vi "SetCellValuesInXLS.vi"() -> ()   [LabVIEW 2013]
uses:
  C:/PhaeronGit/LVNPOI/Resources/NPOI 2.1.1 dotnet2/NPOI.dll
  Resources/NPOI 2.1.1 dotnet2/NPOI.dll
panel:
  in  "File Name":path=path "C:/PhaeronGit/LVNPOI/Scratch/test.xls"
  # "LabVIEW implementation of SetCellValuesInXLS.cs"
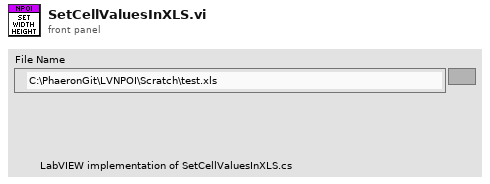
[diagram p1: front panel]
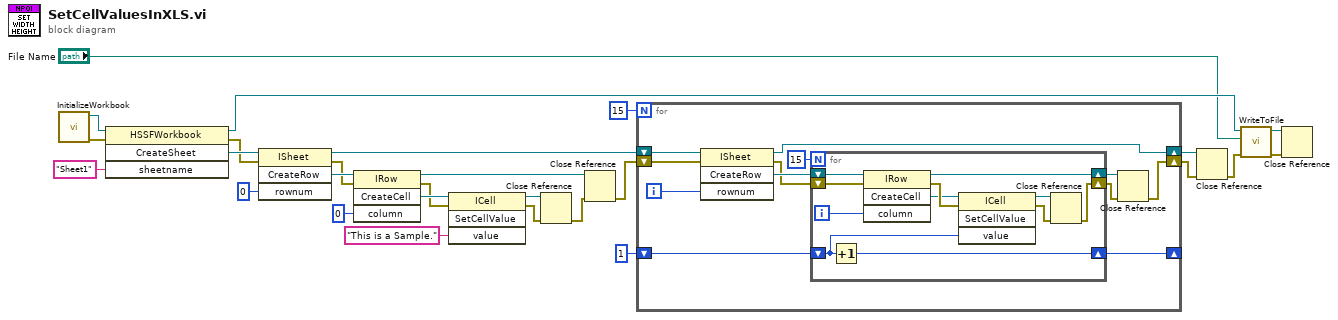
[diagram p0: block diagram]
diagram:
  n1 = call "InitializeWorkbook.vi"() -> ("error out"=w26:errorcluster, "hssfworkbook"=w27:refnum<k24>)  [unwired: 10 in]
  n2 = invoke class="HSSFWorkbook" method="CreateSheet"(reference=w27, error in=w26, "sheetname"="Sheet1") -> (reference out=w25:refnum<k24>, error out=w17:errorcluster, "CreateSheet"=w20:refnum<k24>)  [unwired: 1 in, 1 out]
  n3 = invoke class="ISheet" method="CreateRow"(reference=w20, error in=w17, "rownum"=0) -> (reference out=w6:refnum<k24>, error out=w15:errorcluster, "CreateRow"=w16:refnum<k24>)  [unwired: 1 in, 1 out]
  n4 = invoke class="IRow" method="CreateCell"(reference=w16, error in=w15, "column"=0) -> (reference out=w7:refnum<k24>, error out=w12:errorcluster, "CreateCell"=w13:refnum<k24>)  [unwired: 1 in, 1 out]
  n5 = invoke class="ICell" method="SetCellValue"(reference=w13, error in=w12, "value"="This is a Sample.") -> (reference out=w10:refnum<k24>, error out=w9:errorcluster)  [unwired: 1 in, 2 out]
  n6 = Close Reference(reference=w10, error in (no error)=w9) -> (error out=w8:errorcluster)
  n7 = Close Reference(reference=w7, error in (no error)=w8) -> (error out=w3:errorcluster)
  n8 = for {
    N: 15 -> [_]
    shift-right: [w38] -> w5
    shift-left: w6 -> [w39]
    shift-right: [w29] -> w1
    shift-left: w3 -> [w36]
    shift-right: [w34] -> _
    shift-left: 1 -> [w35]
    i -> [w28]
    n9 = invoke class="ISheet" method="CreateRow"(reference=w39, error in=w36, "rownum"=w28) -> (reference out=w38:refnum<k24>, error out=w31:errorcluster, "CreateRow"=w37:refnum<k24>)  [unwired: 1 in, 1 out]
    n10 = for {
      N: 15 -> [_]
      shift-right: [w44] -> w32
      shift-left: w37 -> [w46]
      shift-right: [w45] -> w34
      shift-left: w35 -> [w41]
      shift-right: [w42] -> w30
      shift-left: w31 -> [w43]
      i -> [w40]
      n11 = Increment(x=w41) -> (x+1=w45:i32)
      n12 = invoke class="IRow" method="CreateCell"(reference=w46, error in=w43, "column"=w40) -> (reference out=w44:refnum<k24>, error out=w48:errorcluster, "CreateCell"=w47:refnum<k24>)  [unwired: 1 in, 1 out]
      n13 = invoke class="ICell" method="SetCellValue"(reference=w47, error in=w48, "value"=w41) -> (reference out=w49:refnum<k24>, error out=w50:errorcluster)  [unwired: 1 in, 2 out]
      n14 = Close Reference(reference=w49, error in (no error)=w50) -> (error out=w42:errorcluster)
    }
    n15 = Close Reference(reference=w32, error in (no error)=w30) -> (error out=w29:errorcluster)
  }
  n16 = Close Reference(reference=w5, error in (no error)=w1) -> (error out=w24:errorcluster)
  n17 = call "WriteToFile.vi"("error in (no error)"=w24, "File Name"="File Name", "hssfworkbook"=w25) -> ("error out"=w21:errorcluster, "hssfworkbook"=w22:refnum<k24>)  [unwired: 7 in]
  n18 = Close Reference(reference=w22, error in (no error)=w21) -> ()  [unwired: 1 out]
